vi "wavemakerdialog.vi"() -> (1 "amplitude (volts)":dbl format="%.2f", 2 "waveform":sgl[](array[numeric]) format="%.2f", 3 "new file path":path)   [LabVIEW 2010]
uses:
  <vilib>/Utility/file.llb/Write To Spreadsheet File (DBL).vi
panel:
  in  "stop":bool
  in  "Get Wave":bool
  in  "solitary wave":T1={"hold (ticks)"=0, "return (ticks)"=1} {"return (ticks)" min=1}
  out "graph":sgl[](graph)
  in  "excursion (cm)":sgl=1.0 min=0 max=12.7 step=1 format="%.2f"
  out "total displacement (cm)":dbl format="%.3f"
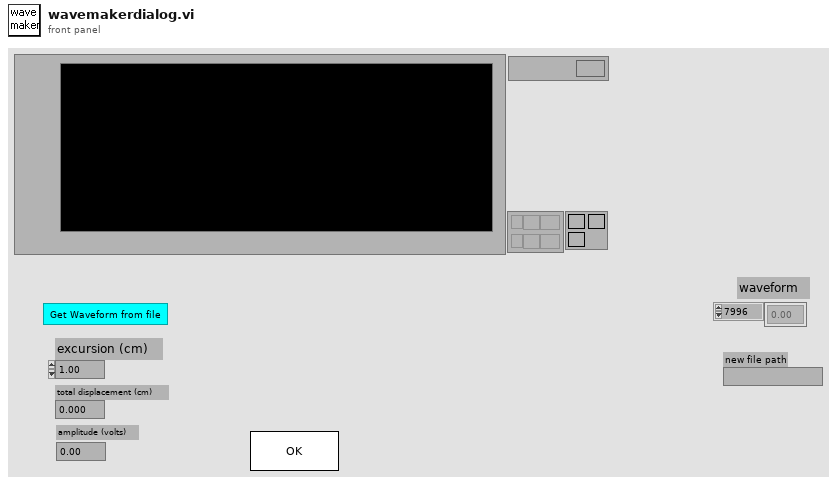
[diagram p1: front panel]
types:
  T1 = cluster{"hold (ticks)":u32, "return (ticks)":u32}
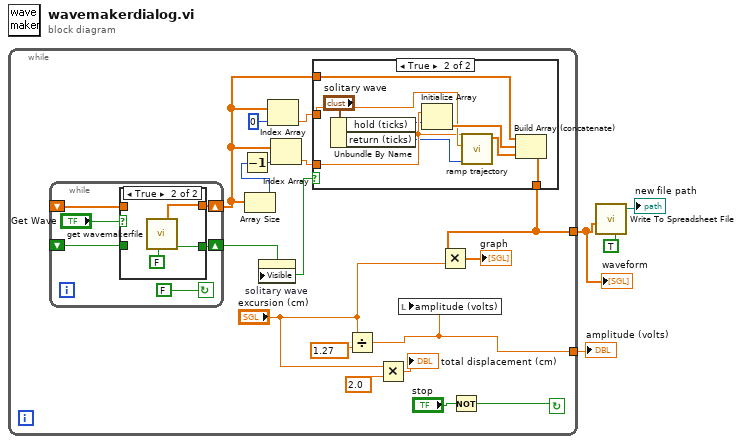
[diagram p0: block diagram]
diagram:
  n1 = while {
    tunnel: [w7] -> w2
    tunnel: [w6] -> w3
    stop <- w20 continue-if-true
    n2 = while {
      shift-left: _ -> [w22]
      shift-right: [w23] -> w9
      shift-left: _ -> [w25]
      shift-right: [w24] -> w18
      stop <- FALSE continue-if-true
      n3 = case shown="True" "Get Wave" {
        tunnel: [w28 w30] -> w24
        tunnel: w25 -> [w28 _]
        tunnel: [w27 w29] -> w23
        tunnel: w22 -> [w27 _]
        frame False {
        }
        frame True {
          n4 = call "get wavemakerfile.vi"("warning"=FALSE) -> ("discontinuities"=w29:bool, "waveform"=w30:sgl[])  [unwired: 8 in, 1 out]
        }
      }
    }
    n5 = Array Size(array=w18) -> (size(s)=w17:i32)
    n6 = Decrement(x=w17) -> (x-1=w16:i32)
    n7 = property on="solitary wave" class="Clust (strict)"("Visible"=w9) -> ()  [unwired: 2 in, 2 out]
    n8 = Index Array(array=w18, index=0) -> (element=w14:sgl)
    n9 = Index Array(array=w18, index=w16) -> (element=w15:sgl)
    n10 = case shown="True" w9 {
      tunnel: w14 -> [_ w36]
      tunnel: w15 -> [_ w35]
      tunnel: w18 -> [w32 w37]
      tunnel: [w32 w38] -> w7
      frame False {
      }
      frame True {
        n11 = Unbundle By Name("solitary wave") -> ("hold (ticks)"=w34:u32, "return (ticks)"=w33:u32)
        n12 = Initialize Array(w35, w34) -> (w40:sgl[])
        n13 = call "ramp trajectory.vi"("points"=w33, "end (volts)"=w36, "start (volts)"=w35) -> ("ramp"=w39:sgl[])  [unwired: 8 in]
        n14 = Build Array (concatenate)(w37, w40, w39) -> (w38:sgl[])
      }
    }
    n15 = Divide(x="excursion (cm)", y=1.27) -> (x/y=w6:dbl)
    n16 = Multiply(x="excursion (cm)", y=2.0) -> (x*y=→"total displacement (cm)":dbl)
    n17 = local write "amplitude (volts)"(w6) -> ()
    n18 = Multiply(x=w7, y="excursion (cm)") -> (x*y=→"graph":sgl[])
    n19 = Not(x="stop") -> (.not. x?=w20:bool)
  }
  "amplitude (volts)" <- w3
  "waveform" <- w2
  n20 = call-poly <vilib>:"Write To Spreadsheet File.vi"("transpose? (no:F)"=TRUE, "1D data"=w2) -> ("new file path (Not A Path if cancelled)"=→"new file path":path)  [unwired: 6 in]
